vi "FGEN-SCOPE.vi"(0 "Device Name":tag="Dev1", 1 "Amplitude":dbl caption="FGEN_Amplitude", 2 "DC Offset":dbl caption="FGEN_DC_Offset", 3 "Frequency":dbl caption="FGEN_Frequency", 4 "Waveform Type":enum16{"Sine", "Triangular", "Square"}(ring) caption="FGEN_Waveform_Type", 5 "Sample Rate (Hz)":dbl=100000.0 caption="SCOPEH_SampleRate" min=0.0 step=1000000.0 format="%#_4p", 6 "Record Length":i32=2000 caption="SCOPEH_RecordLength" min=5 max=75000000 step=1 format="%#.9p", 7 "Acquire":u16(ring)=10178 caption="SCOPEH_Acquire" items=["N Samples"=10178, "Continuously"=10123], 8 "ChA_Source":T3 items=["BNC/Board CH A", "ACH0", "ACH1", "ACH2", "ACH5", "FGEN FUNC_OUT", "FGEN SYNC_OUT", "DMM Voltage"], 9 "ChB_Source":T2 items=["BNC/Board CH B", "ACH0", "ACH1", "ACH2", "ACH5", "FGEN FUNC_OUT", "FGEN SYNC_OUT", "DMM Voltage"], 10 "ChA Coupling":u16(ring) caption="ChA_Coupling" items=["DC", "AC"], 11 "ChB_ Coupling":u16(ring) caption="ChB_Coupling" items=["DC", "AC"], 12 "ChA Range":dbl caption="ChA_Range", 13 "ChB Range":dbl caption="ChB_Range", 14 "ChA Offset":dbl caption="ChA_Offset", 15 "ChB Offset":dbl caption="ChB_Offset", 16 "Trigger Source":u16(ring) caption="SCOPET_Source" items=["Immediate", "TRIGGER", "SYNC_OUT", "CH A", "CH B"], 17 "Trigger Type":u16(ring) caption="SCOPET_Type" items=["Digital", "Analog"], 18 "Slope":i32(ring) caption="SCOPET_Slope" items=["Positive", "Negative"], 19 "Level":dbl caption="SCOPET_Level") -> (20 "Complete?":bool=TRUE, 24 "interleaved array":dbl[](array[numeric]))   [LabVIEW 2010]
uses:
  <instrlib>/NI ELVIS Traditional/NI ELVIS - Scope.llb/ELVIS SCOPE - Channel A Source.ctl
  <instrlib>/NI ELVIS Traditional/NI ELVIS - Scope.llb/ELVIS SCOPE - Channel B Source.ctl
  <vilib>/Analysis/Matrix/Datatypes/RealMatrix.ctl
  Instance           1 18Saved   FGEN-SCOPE .vi
  Instance           4 18Saved   FGEN-SCOPE .vi
  Instance           2 18Saved   FGEN-SCOPE .vi
  Instance           5 18Saved   FGEN-SCOPE .vi
  <vilib>/Analysis/Matrix/Numeric/Conversions/Array To Matrix - RA.vi
  <vilib>/Analysis/Matrix/NI_Matrix.lvlib
panel:
  out "CH A":T1
  out "CH B":T1
  out "Record count":i32
  out "overall scan time (seconds)":dbl
  out "Waveform Graph":dynamicdata(graph)
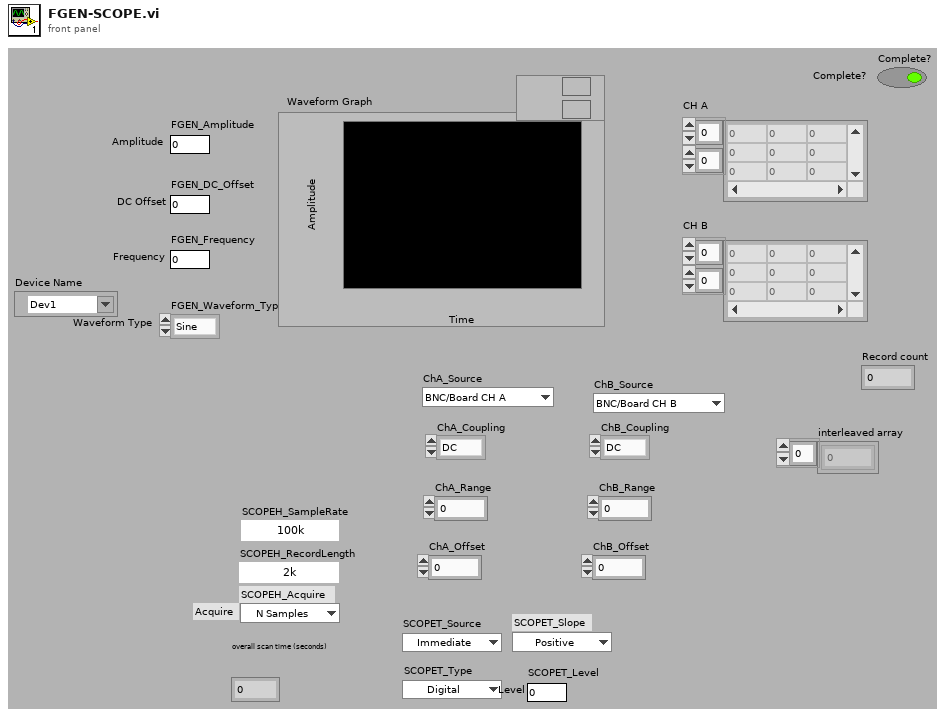
[diagram p1: front panel]
types:
  T1 = typedef "NI_Matrix.lvlib/RealMatrix.ctl" = dbl[][]
  T2 = typedef "ELVIS SCOPE - Channel B Source.ctl" = u16
  T3 = typedef "ELVIS SCOPE - Channel A Source.ctl" = u16
  T4 = cluster{"Trigger Source":u16, "Trigger Type":u16, "Slope":i32, "Level":dbl}
  T5 = cluster{"ChA Range":dbl, "ChA Offset":dbl, "ChA_Source":T3, "ChA Coupling":u16}
  T6 = cluster{"ChB Range":dbl, "ChB Offset":dbl, "ChB_Source":T2, "ChB_ Coupling":u16}
  T7 = cluster{"Sample Rate (Hz)":dbl, "Record Length":i32, "Acquire":u16}
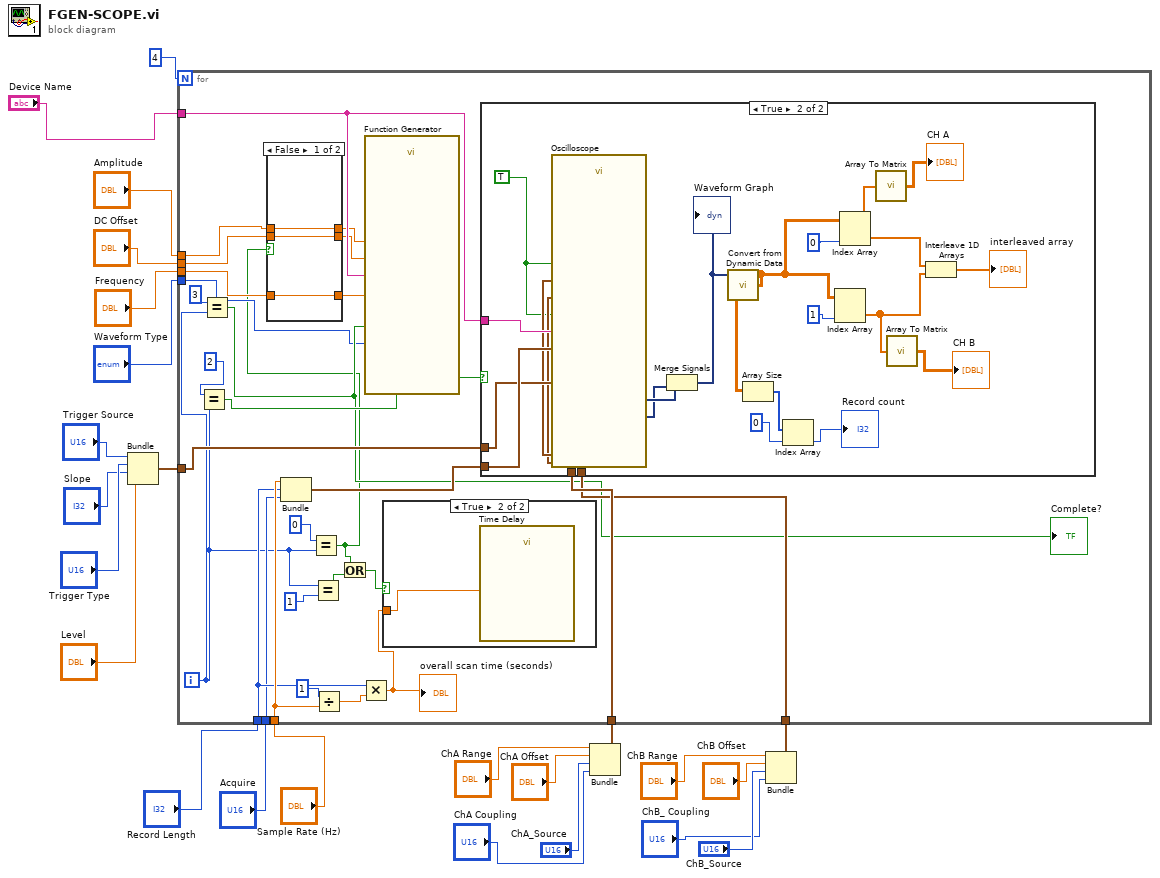
[diagram p0: block diagram]
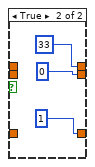
[diagram p2: hidden frame]
diagram:
  n1 = Bundle("Trigger Source"="Trigger Source", "Trigger Type"="Trigger Type", "Slope"="Slope", "Level"="Level") -> (w15:T4)  [unwired: 1 in]
  n2 = Bundle("ChA Range"="ChA Range", "ChA Offset"="ChA Offset", "ChA_Source"="ChA_Source", "ChA Coupling"="ChA Coupling") -> (w10:T5)  [unwired: 1 in]
  n3 = Bundle("ChB Range"="ChB Range", "ChB Offset"="ChB Offset", "ChB_Source"="ChB_Source", "ChB_ Coupling"="ChB_ Coupling") -> (w5:T6)  [unwired: 1 in]
  n4 = for {
    N: 4 -> [_]
    tunnel: "Sample Rate (Hz)" -> [w48]
    tunnel: "Record Length" -> [w47]
    tunnel: "Acquire" -> [w45]
    tunnel: "Device Name" -> [w38]
    tunnel: "Amplitude" -> [w36]
    tunnel: "DC Offset" -> [w34]
    tunnel: "Frequency" -> [w32]
    tunnel: "Waveform Type" -> [w30]
    tunnel: w15 -> [w44]
    tunnel: w10 -> [w43]
    tunnel: w5 -> [w42]
    i -> [w25]
    n5 = Equal?(x=2, y=w25) -> (x = y?=w46:bool)
    n6 = Equal?(x=3, y=w25) -> (x = y?=w37:bool)
    "Complete?" <- w37
    n7 = Bundle("Sample Rate (Hz)"=w48, "Record Length"=w47, "Acquire"=w45) -> (w49:T7)  [unwired: 1 in]
    n8 = Equal?(x=0, y=w25) -> (x = y?=w27:bool)
    n9 = case shown="False" w27 {
      tunnel: w36 -> [w55 _]
      tunnel: [w55 33] -> w35
      tunnel: w34 -> [w54 _]
      tunnel: [w54 0] -> w33
      tunnel: w32 -> [w53 _]
      tunnel: [w53 1] -> w31
      frame False {
      }
      frame True {
      }
    }
    n10 = Equal?(x=w25, y=1) -> (x = y?=w28:bool)
    n11 = Divide(x=1, y=w48) -> (x/y=w50:dbl)
    n12 = Or(x=w27, y=w28) -> (x .or. y?=w26:bool)
    n13 = Multiply(x=w47, y=w50) -> (x*y=w41:dbl)
    "overall scan time (seconds)" <- w41
    n14 = call "Function Generator"("Device Name"=w38, "Stop"=w37, "Frequency (Hz)"=w31, "DC Offset (V)"=w33, "Amplitude (V)"=w35, "Type"=w30) -> ()  [unwired: 12 in, 2 out]
    n15 = case shown="True" w26 {
      tunnel: w41 -> [_ w59]
      frame False {
      }
      frame True {
        n16 = call "Time Delay"("Delay Time (s)"=w59) -> ()  [unwired: 10 in, 1 out]
      }
    }
    n17 = case shown="True" w46 {
      tunnel: w49 -> [_ w79]
      tunnel: w44 -> [_ w78]
      tunnel: w38 -> [_ w76]
      tunnel: w43 -> [_ w62]
      tunnel: w42 -> [_ w61]
      frame False {
      }
      frame True {
        w60 = TRUE
        n18 = call "Oscilloscope"("Device Name"=w76, "Channel A"=w62, "ChA Enable"=w60, "Channel B"=w61, "ChB Enable"=w60, "Trigger"=w78, "Horizontal"=w79) -> ("ELVIS/ChannelA"=w77:dynamicdata, "ELVIS/ChannelB"=w75:dynamicdata)  [unwired: 10 in, 1 out]
        n19 = Merge Signals(w77, w75) -> (w71:dynamicdata)
        "Waveform Graph" <- w71
        n20 = call "Convert from Dynamic Data"("Dynamic Data Type"=w71) -> ("Array"=w64:dbl[][])  [unwired: 3 in]
        n21 = Array Size(array=w64) -> (size(s)=w74:i32[])
        n22 = Index Array(array=w74, index=0) -> (element=→"Record count":i32)
        n23 = Index Array(array=w64, index (col)=1) -> (element=w65:dbl[])  [unwired: 1 in]
        n24 = Index Array(array=w64, index (col)=0) -> (element=w66:dbl[])  [unwired: 1 in]
        n25 = call-poly <vilib>:"Array To Matrix.vi"("Real 1D Array"=w66) -> ("Real Matrix (Column Vector)"=→"CH A":T1)
        n26 = call-poly <vilib>:"Array To Matrix.vi"("Real 1D Array"=w65) -> ("Real Matrix (Column Vector)"=→"CH B":T1)
        n27 = Interleave 1D Arrays(w66, w65) -> (→"interleaved array":dbl[])
      }
    }
  }
